vi "Make from Test Case.vi"(8 "error in (no error)":errorcluster, 10 "LUnit Test Case":refnum<class "LUnit Test Case V2.lvclass">) -> (0 "error out":errorcluster, 3 "LUnit Test Suite V2 out":refnum<class "LUnit Test Suite V2.lvclass">)   [LabVIEW 2020, in "LUnit Test Suite V2.lvclass"]
uses:
  LUnit Test Suite V2.lvclass
  LUnit Test Case/LUnit Test Case V2.lvclass
  C:/Git/astemes-lunit/source/Rewrite Project/Run/Runnable.lvclass
  Result/Type.ctl
  LUnit Test Suite V2.lvclass/LUnit Test Suite V2.ctl
  Result/Result.lvlib
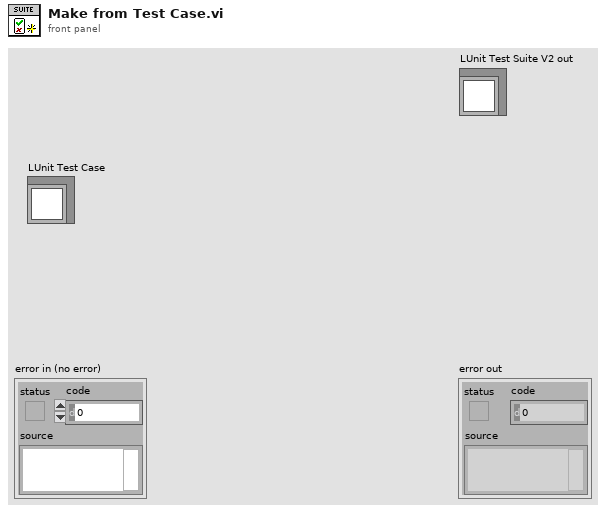
[diagram p1: front panel]
types:
  T1 = typedef "Result.lvlib/Type.ctl" = enum16{"Assertion", "Method", "Case", "Suite"}
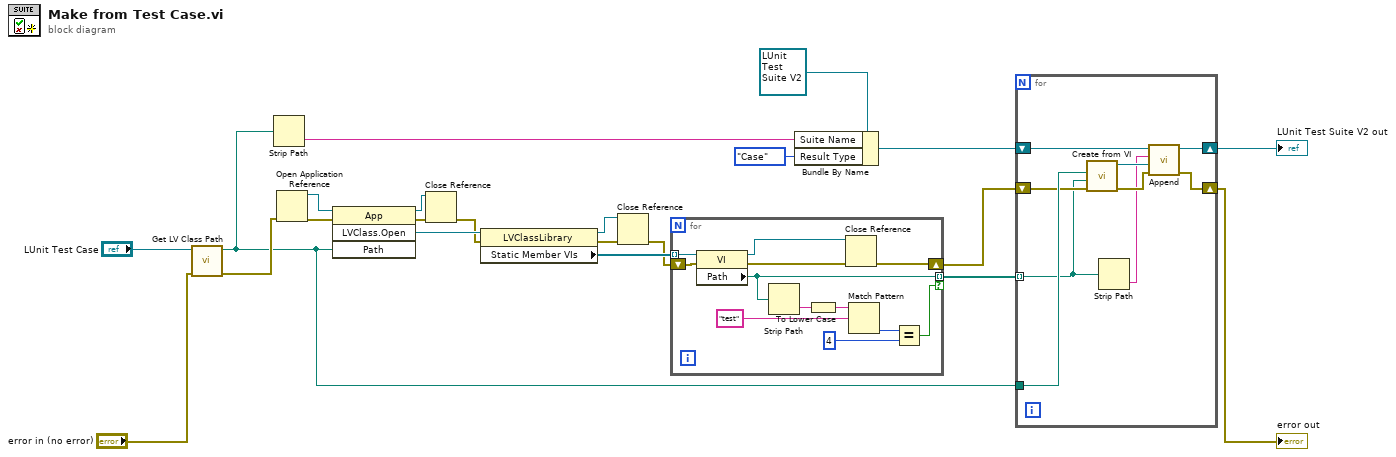
[diagram p0: block diagram]
diagram:
  n1 = call <vilib>:"Get LV Class Path.vi"("error in (no error)"="error in (no error)", "object"="LUnit Test Case") -> ("error out"=w11:errorcluster, "class path"=w4:path)  [unwired: 8 in]
  n2 = Strip Path(path=w4) -> (name=w2:string)  [unwired: 1 out]
  n3 = Open Application Reference(8:w11) -> (0:w19:errorcluster, 3:w20:refnum<vi>)  [unwired: 3 in]
  n4 = invoke class="App" method="LVClass.Open"(reference=w20, error in=w19, "Path"=w4) -> (reference out=w5:refnum<vi>, error out=w17:errorcluster, "LVClass.Open"=w18:refnum<vi>)  [unwired: 1 in, 1 out]
  n5 = Close Reference(reference=w5, error in (no error)=w17) -> (error out=w6:errorcluster)
  n6 = property class="LVClassLibrary"(reference=w18, error in=w6) -> (reference out=w7:refnum<vi>, error out=w10:errorcluster, "Static Member VIs"=w16:refnum<vi>[])
  n7 = Close Reference(reference=w7, error in (no error)=w10) -> (error out=w8:errorcluster)
  n8 = for {
    tunnel: w16 -> [w34] mode=indexing
    tunnel: [w24] -> w15 mode=indexing if=w29
    shift-right: [w26] -> w9
    shift-left: w8 -> [w28]
    n9 = property class="VI"(reference=w34, error in=w28) -> (reference out=w25:refnum<vi>, error out=w27:errorcluster, "Path"=w24:path)
    n10 = Strip Path(path=w24) -> (name=w23:string)  [unwired: 1 out]
    n11 = To Lower Case(string=w23) -> (all lower case string=w32:string)
    n12 = Close Reference(reference=w25, error in (no error)=w27) -> (error out=w26:errorcluster)
    n13 = Match Pattern(string=w32, regular expression="test") -> (offset past match=w31:i32)  [unwired: 1 in, 3 out]
    n14 = Equal?(x=w31, y=4) -> (x = y?=w29:bool)
  }
  n15 = Bundle By Name(cluster=refnum<class "LUnit Test Suite V2.lvclass"> refnum ("LUnit Test Suite V2 in"), "Suite Name"=w2, "Result Type"=Type."Case") -> (w3:refnum<class "LUnit Test Suite V2.lvclass">)
  n16 = for {
    tunnel: w4 -> [w43]
    tunnel: w15 -> [w36] mode=indexing
    shift-right: [w41] -> w13
    shift-left: w3 -> [w42]
    shift-right: [w39] -> w12
    shift-left: w9 -> [w38]
    n17 = call "Create from VI.vi"("error in (no error)"=w38, "Test Method VI Path"=w36, "Test Case LVCLass Path"=w43) -> ("error out"=w40:errorcluster, "LUnit Test Case V2 out"=w37:refnum<class "LUnit Test Case V2.lvclass">)  [unwired: 7 in]
    n18 = Strip Path(path=w36) -> (name=w35:string)  [unwired: 1 out]
    n19 = call "Append.vi"("error in (no error)"=w40, "Runnable"=w37, "Name"=w35, "LUnit Test Suite V2 in"=w42) -> ("error out"=w39:errorcluster, "LUnit Test Suite V2 out"=w41:refnum<class "LUnit Test Suite V2.lvclass">)  [unwired: 6 in]
  }
  "error out" <- w12
  "LUnit Test Suite V2 out" <- w13
